vi "Convert Domain.vi"(8 "Direction":enum16{"Forward", "Backward"}(ring), 11 "Real":dbl[](array[numeric])=[0.2787992127517914, 0.23659680929450513, 31.17904685885661]) -> (3 "Unit":dbl[](array[numeric])=[0.27179336078925975, 0.23227872800692473, 0.5177141669170274])   [LabVIEW 2017]
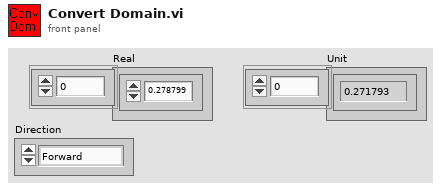
[diagram p1: front panel]
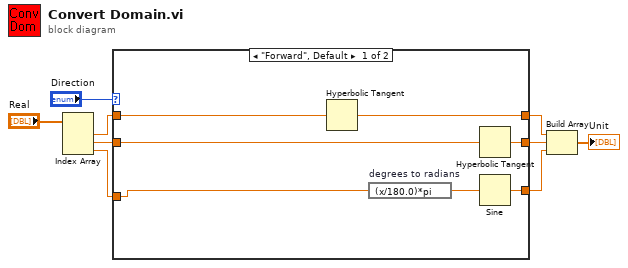
[diagram p0: block diagram]
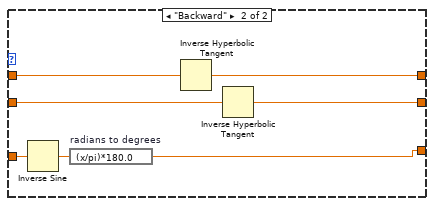
[diagram p2: hidden frame]
diagram:
  n1 = Index Array(array="Real") -> (element #1=w6:dbl, element #2=w7:dbl, element #3=w8:dbl)  [unwired: 3 in]
  n2 = case shown="\"Forward\", Default" "Direction" {
    tunnel: w8 -> [w10 w19]
    tunnel: w7 -> [w16 w21]
    tunnel: w6 -> [w15 w23]
    tunnel: [w14 w17] -> w4
    tunnel: [w13 w20] -> w3
    tunnel: [w12 w22] -> w2
    frame "Forward", Default {
      n3 = Hyperbolic Tangent(1:w15) -> (0:w12:dbl)
      n4 = expression code="(x/180.0)*pi" "degrees to radians"(w10) -> (w11:dbl)
      n5 = Hyperbolic Tangent(1:w16) -> (0:w13:dbl)
      n6 = Sine(x=w11) -> (sin(x)=w14:dbl)
    }
    frame "Backward" {
      n7 = Inverse Sine(1:w19) -> (0:w18:dbl)
      n8 = expression code="(x/pi)*180.0" "radians to degrees"(w18) -> (w17:dbl)
      n9 = Inverse Hyperbolic Tangent(1:w23) -> (0:w22:dbl)
      n10 = Inverse Hyperbolic Tangent(1:w21) -> (0:w20:dbl)
    }
  }
  n11 = Build Array(w2, w3, w4) -> (→"Unit":dbl[])
